vi "Set Scan Active.vi"(8 "error in (no error)":errorcluster caption="에러 입력", 11 "Timeout(Scans)":i32=10000) -> (0 "Error Out":errorcluster caption="에러 출력")   [LabVIEW 2019]
uses:
  Scanengine Status.ctl
  <vilib>/Platform/TimedLoop/XDataNode/timing_clust.ctl
  <vilib>/Platform/TimedLoop/XDataNode/nitl_modes.ctl
  <vilib>/Platform/TimedLoop/XDataNode/wakeup.ctl
  <vilib>/Platform/TimedLoop/XDataNode/XDataNode.xnode
  <vilib>/Platform/TimedLoop/XDataNode/XDNodeRunTimeDep.lvlib
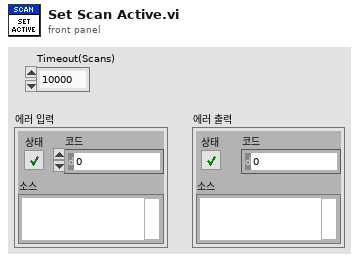
[diagram p1: front panel]
types:
  T1 = typedef "Scanengine Status.ctl" = enum16{"Check Engine State", "Set Config", "Check Config Transition", "Set Active", "Check Active Transition", "Close"}
  T2 = typedef "XDNodeRunTimeDep.lvlib/timing_clust.ctl" = cluster{"Expected End [f-1]":u64, "Actual End [f-1]":u64, "Finished Late? [f-1]":bool, "Expected End [i-1]":u64, "Actual End [i-1]":u64, "Finished Late? [i-1]":bool, "Expected Start [i]":u64, "Actual Start [i]":u64, "Expected Start [f]":u64, "Actual Start [f]":u64, "Source Name":string, "Structure Name":string, "Period":i64, "Deadline":i64, "Offset":i64, "Start":i64, "Priority":i32, "Timeout":i32, "Mode":T3, "Wakeup Reason":T4, "Error":errorcluster, "Source Type":string, "Secondary Source Type":string, "Global End Time":u64, "Global Start Time":u64, "Frame Duration":u64, "Iteration Duration":u64, "Assigned CPU":i32, "I/O Scan Engine Mode":u32}
  T3 = typedef "XDNodeRunTimeDep.lvlib/nitl_modes.ctl" = enum32{"No Change", "Process missed periods, maintain original phase", "Discard missed periods, maintain original phase", "Process missed periods, ignore original phase", "Discard missed periods, ignore original phase"}
  T4 = typedef "XDNodeRunTimeDep.lvlib/wakeup.ctl" = enum32{"Normal", "Aborted", "Asynchronous wakeup", "Timing source error", "Timed loop error", "Timeout"}
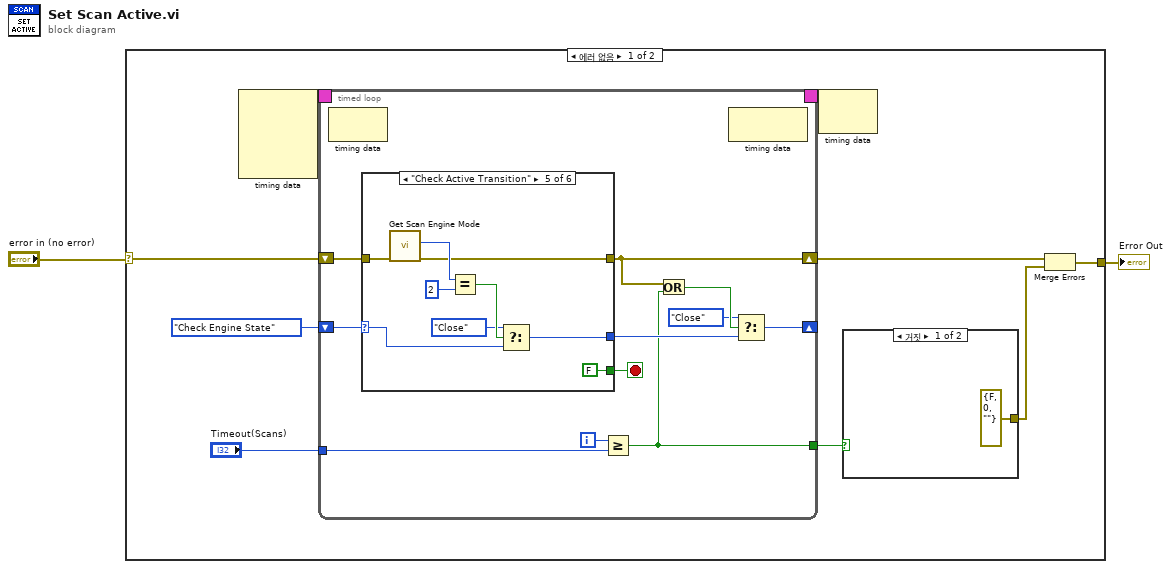
[diagram p0: block diagram]
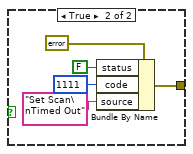
[diagram p2: hidden frame]
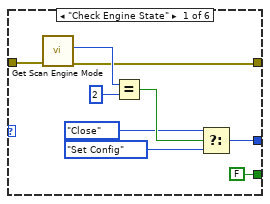
[diagram p3: hidden frame]
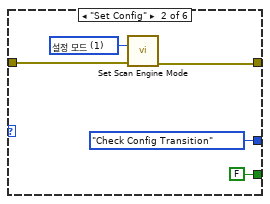
[diagram p4: hidden frame]
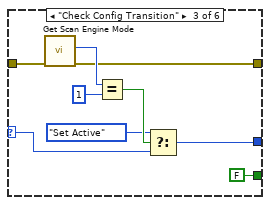
[diagram p5: hidden frame]
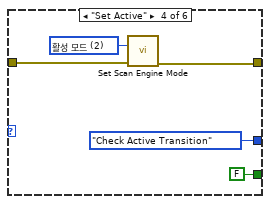
[diagram p6: hidden frame]
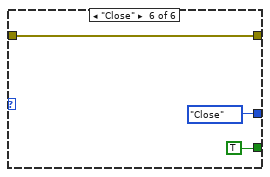
[diagram p7: hidden frame]
diagram:
  n1 = case shown="에러 없음" "error in (no error)" {
    selector: "error in (no error)" -> [w3 w73]
    tunnel: [w4 w73] -> w2
    frame No Error {
      n2 = node-c288() -> (w11:T2)  [unwired: 4 in]
      n3 = timed-loop {
        timing: w11 -> [_]
        timing-out: [_] -> w10
        shift-right: [w21] -> _
        shift-left: Scanengine_Status."Check Engine State" -> [w28]
        shift-right: [w24] -> w6
        shift-left: w3 -> [w27]
        tunnel: "Timeout(Scans)" -> [w20]
        tunnel: [w19] -> w7
        i -> [w26]
        stop <- w25 stop-if-true
        n4 = node-c288() -> ()  [unwired: 1 in, 1 out]
        n5 = case shown="\"Check Active Transition\"" w28 {
          selector: w28 -> [_ _ w46 _ w60 _]
          tunnel: [w34 w40 w49 w54 w63 w68] -> w24
          tunnel: w27 -> [w35 w41 w48 w55 w62 w68]
          tunnel: [w32 Scanengine_Status."Check Config Transition" w45 Scanengine_Status."Check Active Transition" w59 Scanengine_Status."Close"] -> w22
          tunnel: [FALSE FALSE FALSE FALSE FALSE TRUE] -> w25
          frame "Check Engine State" {
            n6 = call <vilib>:"Get Scan Engine Mode.vi"("error in (no error)"=w35) -> ("error out"=w34:errorcluster, "mode"=w37:i32)  [unwired: 9 in]
            n7 = Equal?(x=w37, y=2) -> (x = y?=w33:bool)
            n8 = Select(t=Scanengine_Status."Close", s=w33, f=Scanengine_Status."Set Config") -> (s? t:f=w32:T1)
          }
          frame "Set Config" {
            w42 = 1 items=["설정 모드"=1, "활성 모드"=2] ("mode (Active Mode)")
            n9 = call <vilib>:"Set Scan Engine Mode.vi"("mode (Active Mode)"=w42, "error in (no error)"=w41) -> ("error out"=w40:errorcluster)  [unwired: 13 in]
          }
          frame "Check Config Transition" {
            n10 = call <vilib>:"Get Scan Engine Mode.vi"("error in (no error)"=w48) -> ("error out"=w49:errorcluster, "mode"=w51:i32)  [unwired: 9 in]
            n11 = Equal?(x=w51, y=1) -> (x = y?=w47:bool)
            n12 = Select(t=Scanengine_Status."Set Active", s=w47, f=w46) -> (s? t:f=w45:T1)
          }
          frame "Set Active" {
            w56 = 2 items=["설정 모드"=1, "활성 모드"=2] ("mode (Active Mode)")
            n13 = call <vilib>:"Set Scan Engine Mode.vi"("mode (Active Mode)"=w56, "error in (no error)"=w55) -> ("error out"=w54:errorcluster)  [unwired: 13 in]
          }
          frame "Check Active Transition" {
            n14 = call <vilib>:"Get Scan Engine Mode.vi"("error in (no error)"=w62) -> ("error out"=w63:errorcluster, "mode"=w65:i32)  [unwired: 9 in]
            n15 = Equal?(x=w65, y=2) -> (x = y?=w61:bool)
            n16 = Select(t=Scanengine_Status."Close", s=w61, f=w60) -> (s? t:f=w59:T1)
          }
          frame "Close" {
          }
        }
        n17 = Greater Or Equal?(x=w26, y=w20) -> (x >= y?=w19:bool)
        n18 = Or(x=w24, y=w19) -> (x .or. y?=w23:bool)
        n19 = node-c288() -> ()  [unwired: 1 in, 1 out]
        n20 = Select(t=Scanengine_Status."Close", s=w23, f=w22) -> (s? t:f=w21:T1)
      }
      n21 = node-c288(w10) -> ()  [unwired: 1 out]
      n22 = case shown="거짓" w7 {
        tunnel: [errorcluster {"status"=FALSE, "code"=0, "source"=""} ("error out") w13] -> w5
        frame False {
        }
        frame True {
          n23 = Bundle By Name(cluster=errorcluster {"status"=FALSE, "code"=0, "source"=""} ("error out"), "status"=FALSE, "code"=1111, "source"="Set Scan\nTimed Out") -> (w13:errorcluster)
        }
      }
      n24 = Merge Errors(w6, w5) -> (w4:errorcluster)
    }
    frame Error {
    }
  }
  "Error Out" <- w2
